vi "Write Name.vi"(8 "error in (no error)":errorcluster, 10 "Name":string, 11 "Jedi in":refnum<class "Jedi.lvclass">) -> (0 "error out":errorcluster, 3 "Jedi out":refnum<class "Jedi.lvclass">)   [LabVIEW 2020, in "Jedi.lvclass"]
uses:
  Jedi.lvclass
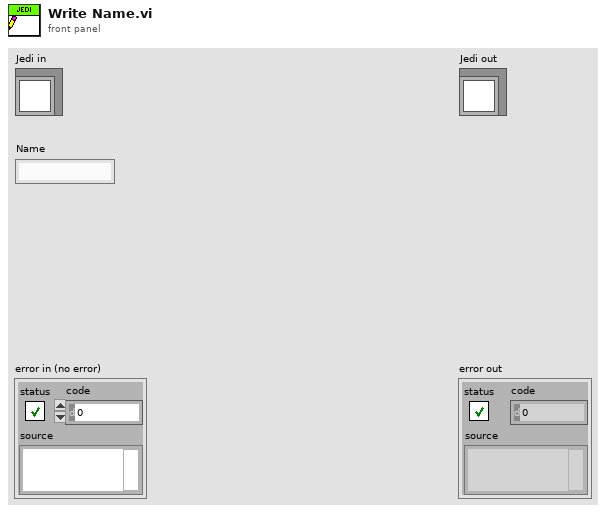
[diagram p1: front panel]
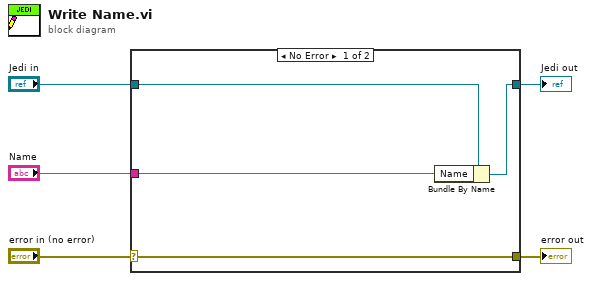
[diagram p0: block diagram]
diagram:
  n1 = case shown="No Error" "error in (no error)" {
    selector: "error in (no error)" -> [w9 w10]
    tunnel: [w9 w10] -> w4
    tunnel: [w7 w11] -> w2
    tunnel: "Jedi in" -> [w8 w11]
    tunnel: "Name" -> [w6 _]
    frame No Error {
      n2 = Bundle By Name(cluster=w8, "Name"=w6) -> (w7:refnum<class "Jedi.lvclass">)
    }
    frame Error {
    }
  }
  "error out" <- w4
  "Jedi out" <- w2
